vi "Climber_Determiner.vi"   [LabVIEW 2020]
uses:
  Climber_Control_States.ctl
  Globals/Climber_Globals.vi
types:
  T1 = typedef "Climber_Control_States.ctl" = enum16{"No-Op", "Manual_%Vbus", "Climbing_Sequence"}
  T2 = typedef "Climber_Cluster.ctl" = cluster{"Control_State":T1, "Outer_Arm_Pivot_Throttle":dbl, "Outer_Arm_Elevator_Throttle":dbl, "Inner_Arm_Pivot_Throttle":dbl, "Enable_Climber_Sequence":bool, "Release_Outer_Pivot_Arm_Brake?":bool}
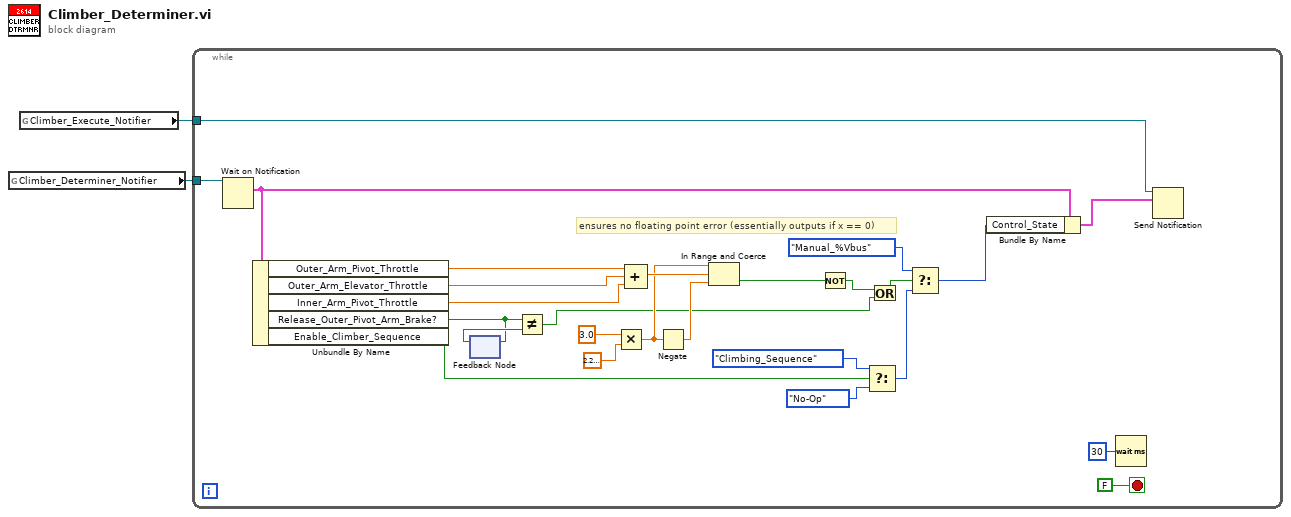
[diagram p0: block diagram]
diagram:
  n1 = global read "Climber_Globals.vi" "Climber_Determiner_Notifier"() -> (w2:refnum<notifier>)
  n2 = global read "Climber_Globals.vi" "Climber_Execute_Notifier"() -> (w1:refnum<notifier>)
  n3 = while {
    tunnel: w2 -> [w28]
    tunnel: w1 -> [w21]
    stop <- FALSE stop-if-true
    # "ensures no floating point error (essentially outputs if x == 0)"
    n4 = Wait on Notification(notifier=w28) -> (notification=w12:T2)  [unwired: 3 in, 3 out]
    n5 = Unbundle By Name(w12) -> ("Outer_Arm_Pivot_Throttle"=w25:dbl, "Outer_Arm_Elevator_Throttle"=w24:dbl, "Inner_Arm_Pivot_Throttle"=w23:dbl, "Release_Outer_Pivot_Arm_Brake?"=w6:bool, "Enable_Climber_Sequence"=w8:bool)
    n6 = feedback-in #1(w6) -> ()
    n7 = feedback #1() -> (w7:bool)  [unwired: 1 in]
    n8 = Not Equal?(x=w6, y=w7) -> (x != y?=w4:bool)
    n9 = Multiply(x=3.0, y=2.220446049250313e-16) -> (x*y=w9:dbl)
    n10 = Compound Arithmetic op=ADD(w25, w24, w23) -> (w20:dbl)
    n11 = Negate(x=w9) -> (-x=w19:dbl)
    n12 = In Range and Coerce(upper limit=w9, x=w20, lower limit=w19) -> (In Range?=w18:bool)  [unwired: 1 out]
    n13 = Not(x=w18) -> (.not. x?=w5:bool)
    n14 = Select(t=Climber_Control_States."Climbing_Sequence" ("Control_State"), s=w8, f=Climber_Control_States."No-Op" ("Control_State")) -> (s? t:f=w14:T1)
    n15 = Or(x=w5, y=w4) -> (x .or. y?=w3:bool)
    n16 = Select(t=Climber_Control_States."Manual_%Vbus" ("Control_State"), s=w3, f=w14) -> (s? t:f=w13:T1)
    n17 = Bundle By Name(cluster=w12, "Control_State"=w13) -> (w22:T2)
    n18 = Wait (ms)(milliseconds to wait=u32 30) -> ()  [unwired: 1 out]
    n19 = Send Notification(notification=w22, notifier=w21) -> ()  [unwired: 1 in, 2 out]
  }
